vi "Check Output Status.vi"(0 "CS in":refnum<class "CS Emulation.lvclass">, 1 "I0":T1 {"Current" min=0.0}, 2 "I1":T1 {"Current" min=0.0}, 3 "I2":T1 {"Current" min=0.0}, 4 "I3":T1 {"Current" min=0.0}, 5 "error in (no error)":errorcluster, 6 "Ranges":u8 max=3 format="%08b", 10 "BoardNum":u32, 12 "Force check":bool) -> (14 "CS out":refnum<class "CS Emulation.lvclass">, 15 "I1 out":T1 {"Current" min=0.0}, 16 "I0 out":T1 {"Current" min=0.0}, 17 "I2 out":T1 {"Current" min=0.0}, 18 "I3 out":T1 {"Current" min=0.0}, 19 "error out":errorcluster)   [LabVIEW 2016, in "CS Emulation.lvclass"]
uses:
  Lib.llb/CS Emulation.lvclass
  Lib.llb/CS Data.ctl
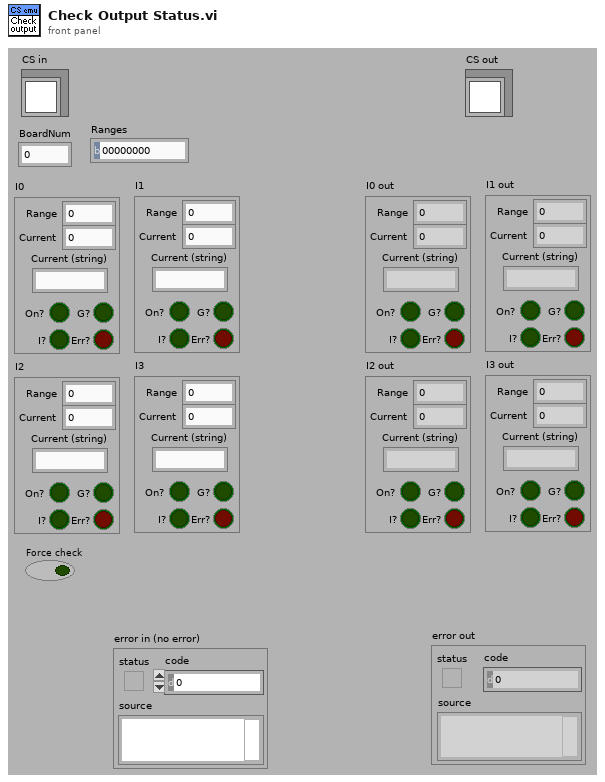
[diagram p1: front panel]
types:
  T1 = typedef "CS Data.ctl" = cluster{"Range":u8, "Current":dbl, "Current (string)":string, "On?":bool, "G?":bool, "I?":bool, "Err?":bool}
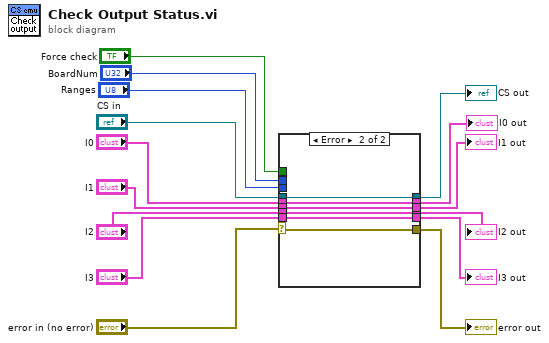
[diagram p0: block diagram]
diagram:
  n1 = case shown="Error" "error in (no error)" {
    selector: "error in (no error)" -> [w16 w22]
    tunnel: "CS in" -> [w21 w27]
    tunnel: "I0" -> [w20 w26]
    tunnel: "I1" -> [w19 w25]
    tunnel: "I2" -> [w18 w24]
    tunnel: "I3" -> [w17 w23]
    tunnel: [w21 w27] -> w10
    tunnel: [w18 w24] -> w9
    tunnel: [w17 w23] -> w8
    tunnel: [w16 w22] -> w7
    tunnel: [w20 w26] -> w6
    tunnel: [w19 w25] -> w5
    tunnel: "Ranges" -> [_ _]
    tunnel: "BoardNum" -> [_ _]
    tunnel: "Force check" -> [_ _]
    frame No Error {
    }
    frame Error {
    }
  }
  "error out" <- w7
  "I1 out" <- w5
  "I3 out" <- w8
  "I2 out" <- w9
  "I0 out" <- w6
  "CS out" <- w10
